vi "ziTC2ENBW.vi"(2 "Order (1)":i32=1, 3 "TC (s)":dbl) -> (0 "Factor":dbl, 1 "ENBW (Hz)":dbl)   [LabVIEW 2009, in "Zurich Instruments LabOne.lvlib"]
doc: "---Obsolete---\nConvert a timeconstant value and order value to the effective equivalent power bandwidth.\n\n<B>Order (1)</B> range: 1 to 8"
uses:
  <instrlib>/Zurich Instruments LabOne/Zurich Instruments LabOne.lvlib
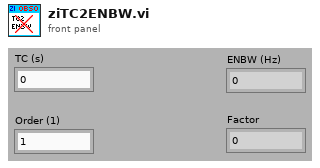
[diagram p1: front panel]
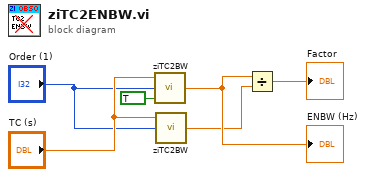
[diagram p0: block diagram]
diagram:
  n1 = call <instrlib>:"ziTC2BW.vi"("Eq BW (F)"=TRUE ("Eq BW"), "Order (1)"="Order (1)", "TC (s)"="TC (s)") -> ("BW (Hz)"=w3:dbl)
  "ENBW (Hz)" <- w3
  n2 = call <instrlib>:"ziTC2BW.vi"("Order (1)"="Order (1)", "TC (s)"="TC (s)") -> ("BW (Hz)"=w2:dbl)  [unwired: 1 in]
  n3 = Divide(x=w3, y=w2) -> (x/y=→"Factor":dbl)
